vi "ConvertBooleanToSCPIValue.vi"(11 "Boolean":bool) -> (3 "SCPI Value":string)   [LabVIEW 2010, in "Keithley-6482-Visa.lvlib"]
uses:
  <instrlib>/lib-labview-8.6-export/Keithley-6482-Visa.lvlib
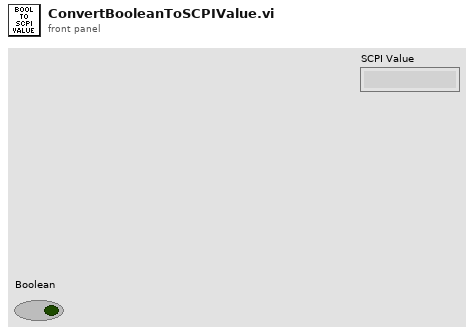
[diagram p1: front panel]
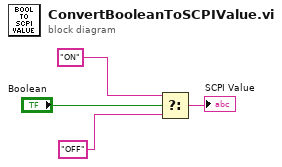
[diagram p0: block diagram]
diagram:
  n1 = Select(t="ON", s="Boolean", f="OFF") -> (s? t:f=→"SCPI Value":string)
